vi "Search User (SubVI).vi"(10 "SelectedUserName":string, 11 "User Info Array in":string[][](array[string])) -> (3 "index of element":i32)   [LabVIEW 2021]
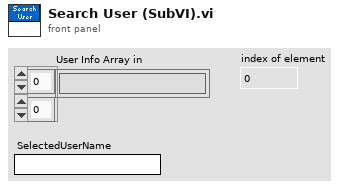
[diagram p1: front panel]
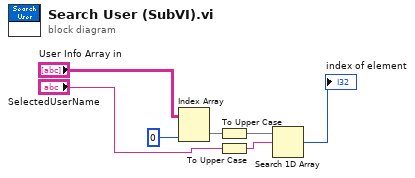
[diagram p0: block diagram]
diagram:
  n1 = Index Array(array="User Info Array in", index (col)=0 ("disabled index (col)")) -> (element=w2:string[])  [unwired: 1 in]
  n2 = To Upper Case(1:w2) -> (0:w3:string[])
  n3 = To Upper Case(1:"SelectedUserName") -> (0:w5:string)
  n4 = Search 1D Array(1D array=w3, element=w5) -> (index of element=→"index of element":i32)  [unwired: 1 in]
